vi "08.1 e 08.2 Groups of Data.vi"() -> ()   [LabVIEW 2019]
panel:
  out "Waveform Graph 2":waveform(dbl)[](graph)
  in  "Waveform Array":waveform(dbl)[](array[waveform])
  out "dt":dbl
  out "Y":dbl[](array[numeric])
  out "attributes":variant
  in  "Waveform":waveform(dbl)
  out "Waveform Graph":dbl[][](graph)
  in  "Array":dbl[][](array[numeric])
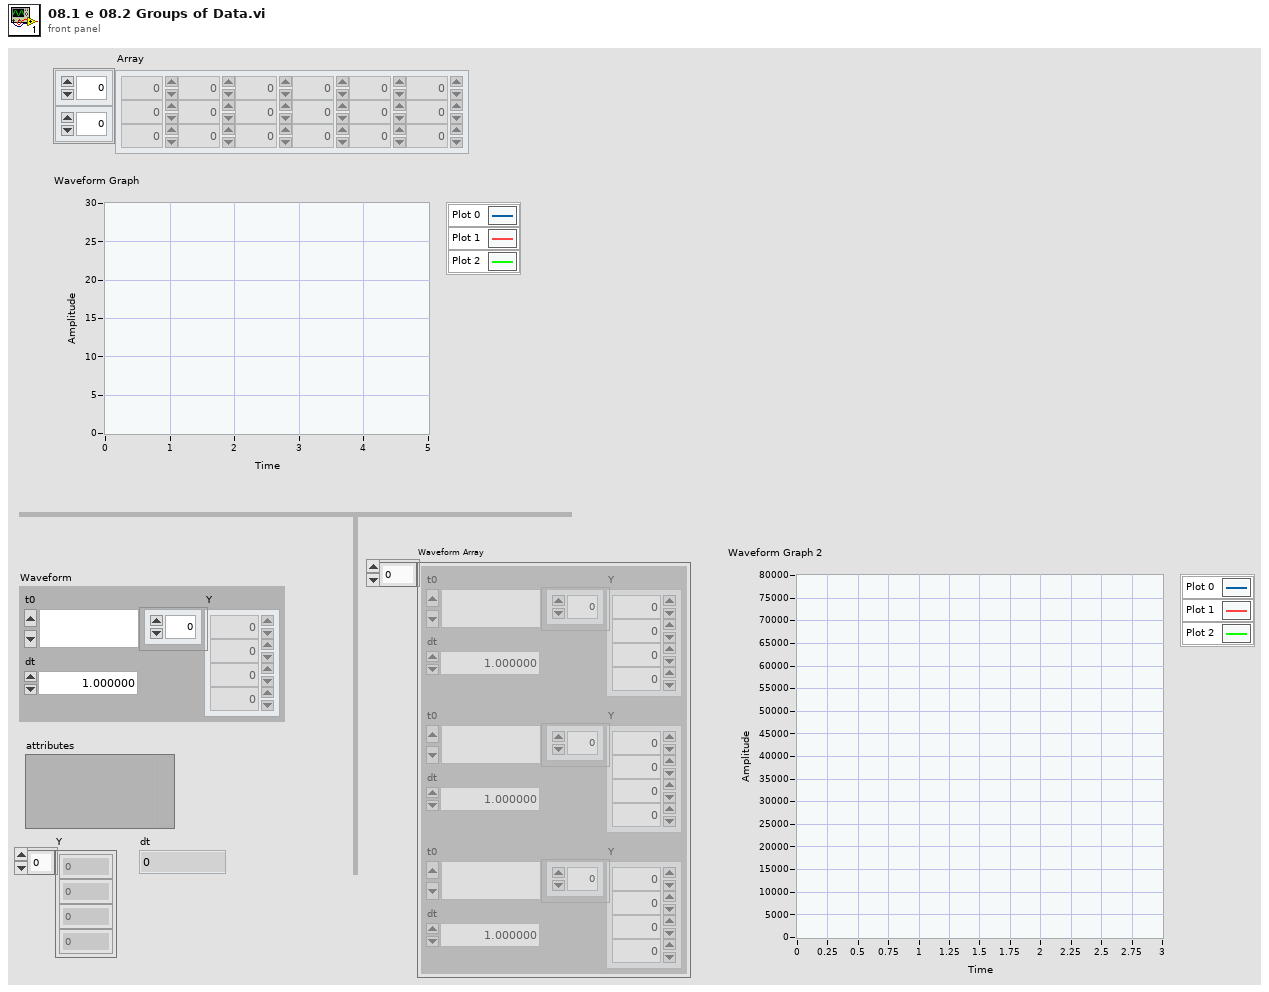
[diagram p1: front panel]
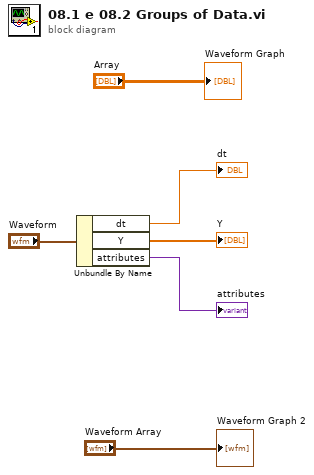
[diagram p0: block diagram]
diagram:
  n1 = Unbundle By Name("Waveform") -> ("dt"=→"dt":dbl, "Y"=→"Y":dbl[], "attributes"=→"attributes":variant)
  "Waveform Graph" <- "Array"
  "Waveform Graph 2" <- "Waveform Array"
